vi "test Get-Set-Get Parameters Configuration File.vi"(8 "error in":errorcluster, 11 "TestCase in":refnum<class "Scripting.lvclass">) -> (0 "error out":errorcluster, 3 "TestCase out":refnum<class "Scripting.lvclass">)   [LabVIEW 2020, in "Scripting.lvclass"]
uses:
  Scripting.lvclass
  <vilib>/addons/_JKI Toolkits/VI Tester/TestCase.llb/TestCase.lvclass
  Scripting/AIM MIL-STD-1553 Scripting.lvlib
  <vilib>/NI/VeriStand Custom Device Testing Tools/VeriStandTestUtilities/VeriStandTestUtilities.lvlib
  C:/Program Files (x86)/National Instruments/LabVIEW 2020/vi.lib/addons/_JKI Toolkits/VI Tester/TestCase.llb/TestCase.lvclass
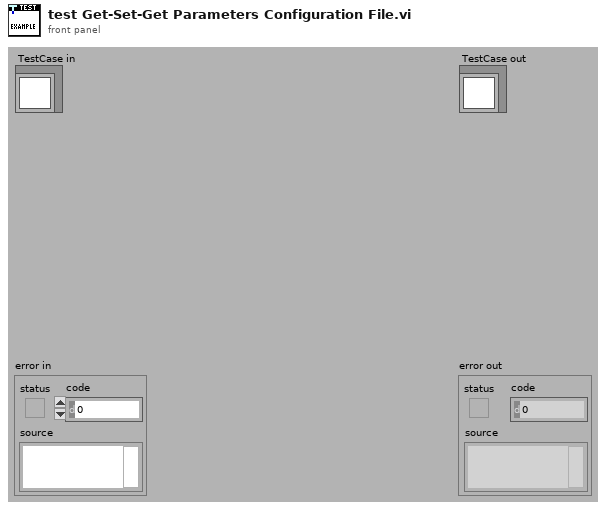
[diagram p1: front panel]
types:
  T1 = typedef "Custom Device API.lvlib/Custom Device Item Ref.ctl" = u64
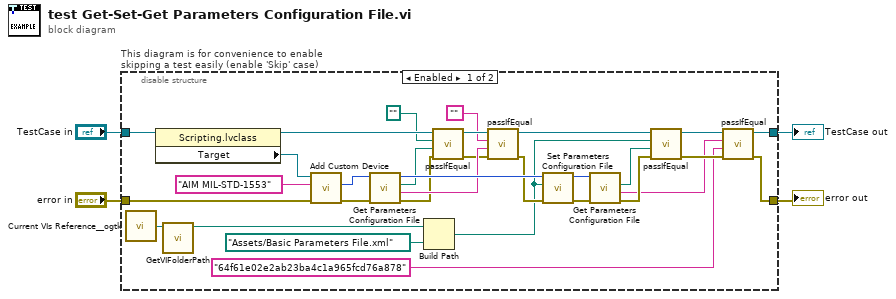
[diagram p0: block diagram]
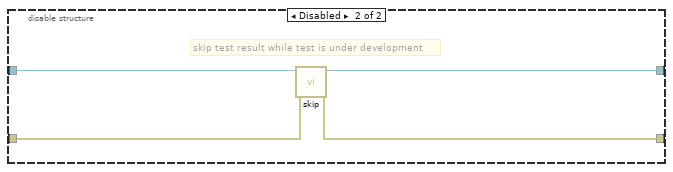
[diagram p2: hidden frame]
diagram:
  n1 = disable-structure "This diagram is for convenience to enable skipping a test easily (enable 'Skip' case)" shown="Enabled" {
    disable-tunnel: "TestCase in" -> [w33 w39]
    disable-tunnel: [w11 w37] -> w1
    disable-tunnel: [w10 w38] -> w3
    disable-tunnel: "error in" -> [w35 w36]
    frame Enabled {
      n2 = call <userlib>:"Current VIs Reference__ogtk.vi"() -> ("Current VI's reference"=w26:refnum<vi>)  [unwired: 5 in]
      n3 = property class="Scripting.lvclass"(reference=w33) -> (reference out=w31:refnum<class "Scripting.lvclass">, "Target"=w32:refnum<k24>)  [unwired: 1 in, 1 out]
      n4 = call <vilib>:"GetVIFolderPath.vi"("VI Reference in"=w26) -> ("VI Folder Path out"=w27:path)  [unwired: 9 in, 1 out]
      n5 = call "Add Custom Device.vi"("error in"=w35, "custom device name"="AIM MIL-STD-1553" ("name"), "target"=w32) -> ("error out"=w29:errorcluster, "custom device"=w30:T1)  [unwired: 6 in, 1 out]
      n6 = call "Get Parameters Configuration File.vi"("error in"=w29, "custom device"=w30) -> ("error out"=w19:errorcluster, "MD5 checksum"=w20:string, "parameters configuration file"=w22:path, "custom device out"=w24:T1)  [unwired: 6 in]
      n7 = Build Path(base path=w27, name or relative path=path "Assets/Basic Parameters File.xml" ("hardware configuration file path")) -> (appended path=w8:path)
      n8 = call-dynamic "passIfEqual.vi"("error in (no error)"=w19, "y"=w22, "x"=path "", "TestCase in"=w31) -> ("error out"=w17:errorcluster, "TestCase out"=w18:refnum<class "Scripting.lvclass">)  [unwired: 6 in]
      n9 = call-dynamic "passIfEqual.vi"("error in (no error)"=w17, "y"=w20, "x"="", "TestCase in"=w18) -> ("error out"=w16:errorcluster, "TestCase out"=w15:refnum<class "Scripting.lvclass">)  [unwired: 6 in]
      n10 = call "Set Parameters Configuration File.vi"("error in"=w16, "parameters configuration file path"=w8, "custom device"=w24) -> ("error out"=w28:errorcluster, "custom device out"=w23:T1)  [unwired: 7 in]
      n11 = call "Get Parameters Configuration File.vi"("error in"=w28, "custom device"=w23) -> ("error out"=w14:errorcluster, "MD5 checksum"=w6:string, "parameters configuration file"=w9:path)  [unwired: 6 in, 1 out]
      n12 = call-dynamic "passIfEqual.vi"("error in (no error)"=w14, "y"=w9, "x"=w8, "TestCase in"=w15) -> ("error out"=w13:errorcluster, "TestCase out"=w12:refnum<class "Scripting.lvclass">)  [unwired: 6 in]
      n13 = call-dynamic "passIfEqual.vi"("error in (no error)"=w13, "y"="64f61e02e2ab23ba4c1a965fcd76a878" ("MD5 checksum"), "x"=w6, "TestCase in"=w12) -> ("error out"=w10:errorcluster, "TestCase out"=w11:refnum<class "Scripting.lvclass">)  [unwired: 6 in]
    }
    frame Disabled {
      # "skip test result while test is under development"
      n14 = call <vilib>:"skip.vi"("error in (no error)"=w36, "TestCase in"=w39) -> ("error out"=w38:errorcluster, "TestCase out"=w37:refnum<class "Scripting.lvclass">)  [unwired: 8 in]
    }
  }
  "error out" <- w3
  "TestCase out" <- w1
